vi "Config 34420 - 4wireres.vi"(1 "error IN":errorcluster, 2 "Address 34420 (default: 13)":string="13") -> (0 "error out":errorcluster)   [LabVIEW 2014]
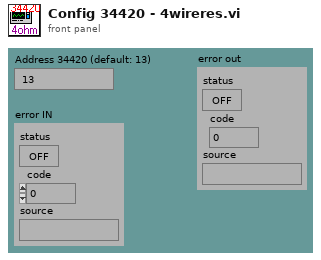
[diagram p1: front panel]
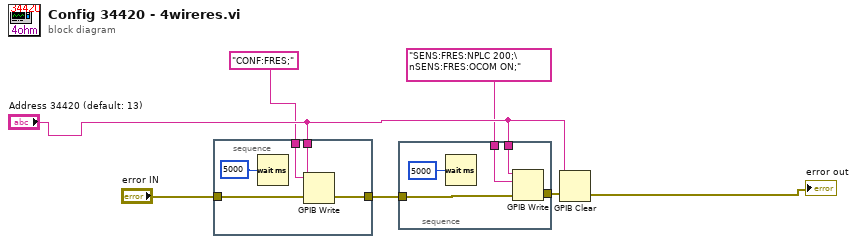
[diagram p0: block diagram]
diagram:
  n1 = stacked-sequence {
    tunnel: "Address 34420 (default: 13)" -> [w12]
    tunnel: "CONF:FRES;" ("Substring") -> [w11]
    tunnel: "error IN" -> [w10]
    tunnel: [w9] -> w1
    frame #0 {
      n2 = Wait (ms)(milliseconds to wait=u32 5000) -> ()  [unwired: 1 out]
      n3 = GPIB Write(0:w12, 1:w11, 3:w10) -> (6:w9:errorcluster)  [unwired: 2 in, 1 out]
    }
  }
  n4 = stacked-sequence {
    tunnel: "Address 34420 (default: 13)" -> [w17]
    tunnel: [w16] -> w5
    tunnel: "SENS:FRES:NPLC 200;\nSENS:FRES:OCOM ON;" ("data") -> [w15]
    tunnel: w1 -> [w14]
    frame #0 {
      n5 = Wait (ms)(milliseconds to wait=u32 5000) -> ()  [unwired: 1 out]
      n6 = GPIB Write(0:w17, 1:w15, 3:w14) -> (6:w16:errorcluster)  [unwired: 2 in, 1 out]
    }
  }
  n7 = GPIB Clear(2:w5, 3:"Address 34420 (default: 13)") -> (0:→"error out":errorcluster)  [unwired: 1 out]
